vi "ni_move.vi"(6 "Axis enable":bool[](array[boolean])=[TRUE, TRUE, TRUE, TRUE], 8 "error in":errorcluster, 9 "Axis positions":dbl[](array[numeric])=[0.0, 0.0, 0.0, 0.0], 10 "Absolute":bool=TRUE) -> (0 "error out":errorcluster)   [LabVIEW 2011]
uses:
  <vilib>/Motion/FlexMotion/CustomControls/CustomControls.llb/AxisOrVectorSpaceControl To Control.flx
  <vilib>/Motion/FlexMotion/CustomControls/CustomControls.llb/AxisOrVectorSpace To Configure.flx
  <vilib>/Motion/FlexMotion/FunctionsVIs/StartStopMotion.llb/Start Motion (8 axes).flx
  <vilib>/Motion/FlexMotion/FunctionsVIs/Trajectory.llb/Wait for Move Complete (8 axes).flx
panel:
  in  "Timeout":u32=60000
  # "The purposes of axis enable is to allow a subset of axes to be driven in absolute position mode without changing (or knowing) the positions of the other axes.   Being disabled just means that we don't want to move that axis, not that we want it powered down."
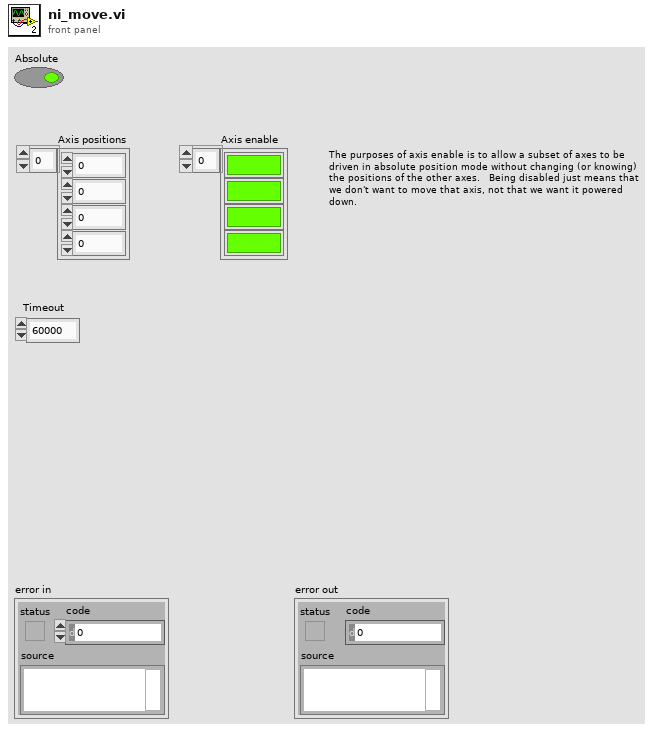
[diagram p1: front panel]
types:
  T1 = typedef "Board Id" = u8
  T2 = enum16{"Absolute Position", "Relative Position", "Velocity", "Relative to Cap Pos", "Modulus Position", "Absolute Contouring", "Relative Contouring"}
  T3 = typedef "AxisOrVectorSpaceControl To Control.flx" = u16
  T4 = typedef "AxisOrVectorSpace To Configure.flx" = u16
  T5 = typedef "Resource Out (Enum).flx" = u16
  T6 = typedef "Bd Id Out" = u8
  T7 = cluster{"Axis enable[0]":bool, "Axis enable[1]":bool, "Axis enable[2]":bool, "Axis enable[3]":bool, "Axis enable[4]":bool, "Axis enable[5]":bool, "Axis enable[6]":bool, "Axis enable[7]":bool}
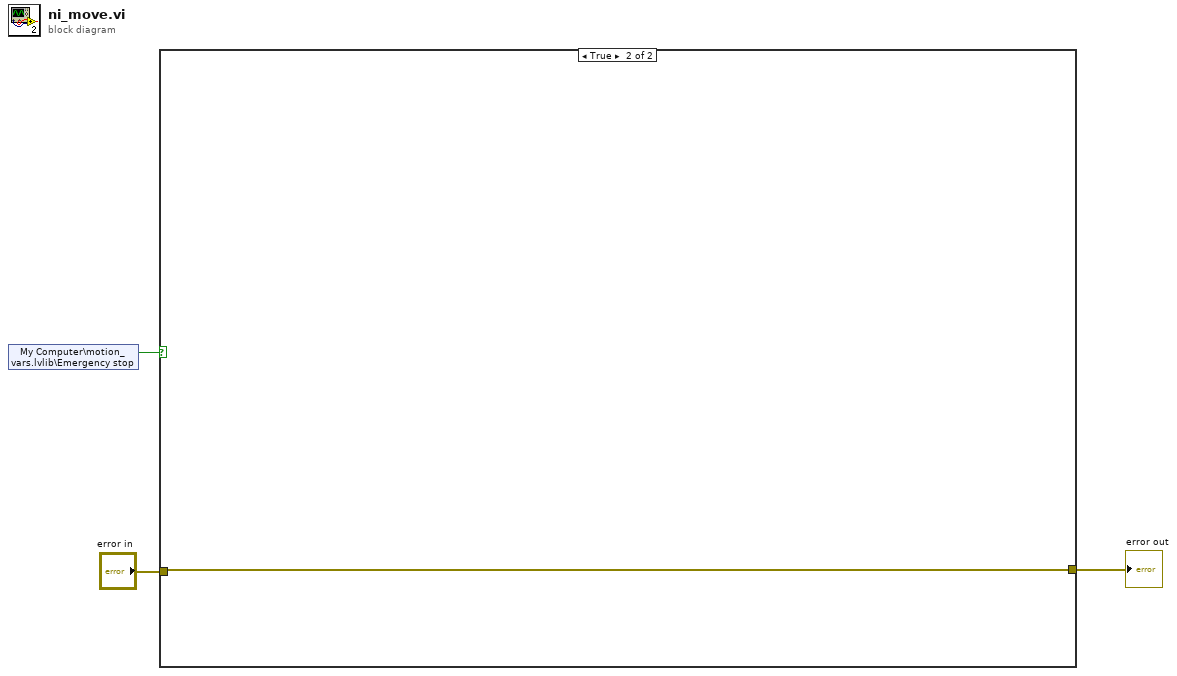
[diagram p0: block diagram]
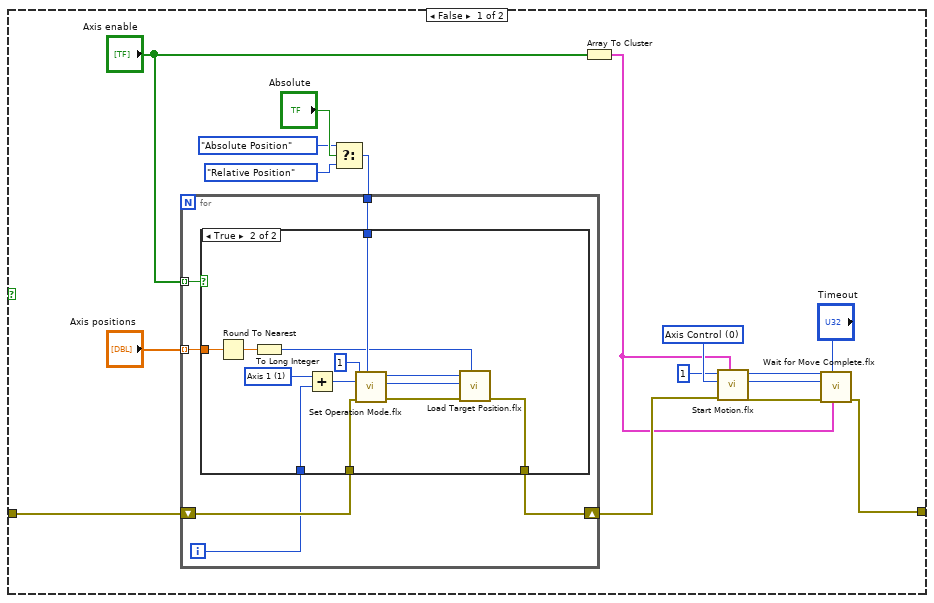
[diagram p2: hidden frame]
diagram:
  n1 = shared-variable "My Computer\\motion_vars.lvlib\\Emergency stop"() -> (w1:bool)  [unwired: 1 in, 1 out]
  n2 = case shown="True" w1 {
    tunnel: "error in" -> [w18 w40]
    tunnel: [w7 w40] -> w2
    frame False {
      w11 = T3 0 items=["Axis Control"=0, "Axis 1"=1, "Axis 2"=2, "Axis 3"=3, "Axis 4"=4, "Axis 5"=5, "Axis 6"=6, "Axis 7"=7, "Axis 8"=8, "Vector Space Control"=16, "Vector Space 1"=17, "Vector Space 2"=18, "Vector Space 3"=19, "Vector Space 4"=20] ("Axis or Vector Space")
      n3 = Select(t=T2."Absolute Position" ("Position Mode (Absolute)"), s="Absolute", f=T2."Relative Position" ("Position Mode (Absolute)")) -> (s? t:f=w15:T2)
      n4 = for {
        tunnel: "Axis enable" -> [w23] mode=indexing
        tunnel: "Axis positions" -> [w22] mode=indexing
        shift-right: [w21] -> w12
        shift-left: w18 -> [w25]
        tunnel: w15 -> [w24]
        i -> [w20]
        n5 = case shown="True" w23 {
          tunnel: w25 -> [w26 w37]
          tunnel: w20 -> [_ w36]
          tunnel: w24 -> [_ w35]
          tunnel: w22 -> [_ w31]
          tunnel: [w26 w28] -> w21
          frame False {
          }
          frame True {
            w39 = T4 1 items=["Axis 1"=1, "Axis 2"=2, "Axis 3"=3, "Axis 4"=4, "Axis 5"=5, "Axis 6"=6, "Axis 7"=7, "Axis 8"=8, "Vector Space 1"=17, "Vector Space 2"=18, "Vector Space 3"=19, "Vector Space 4"=20] ("Axis or Vector Space")
            n6 = Round To Nearest(number=w31) -> (nearest integer value=w30:dbl)
            n7 = To Long Integer(number=w30) -> (32bit integer=w29:i32)
            n8 = Add(x=w39, y=w36) -> (x+y=w38:i32)
            n9 = call <vilib>:"Set Operation Mode.flx"("Position Mode (Absolute)"=w35, "error in (no error)"=w37, "Axis or Vector Space"=w38, "Board ID"=T1 1) -> ("error out"=w32:errorcluster, "Resource Output"=w33:T5, "Bd ID Out"=w34:T6)  [unwired: 2 in]
            n10 = call <vilib>:"Load Target Position.flx"("Target Position (0)"=w29, "error in (no error)"=w32, "Axis"=w33, "Board ID"=w34) -> ("error out"=w28:errorcluster)  [unwired: 3 in, 2 out]
          }
        }
      }
      n11 = Array To Cluster(array="Axis enable") -> (cluster=w10:T7)
      n12 = call-poly <vilib>:"Start Motion.flx"("Axis/VS Map (Disabled)"=w10, "error in (no error)"=w12, "Axis or Vector Space"=w11, "Board ID"=T1 1) -> ("error out"=w8:errorcluster, "Resource Output"=w9:T5, "Bd ID Out"=w5:T6)  [unwired: 2 in]
      n13 = call-poly <vilib>:"Wait for Move Complete.flx"("Axis/VS Map (Disabled)"=w10, "Timeout (10000 ms)"="Timeout", "error in (no error)"=w8, "Axis or Vector Space"=w9, "Board ID"=w5) -> ("error out"=w7:errorcluster)  [unwired: 3 in, 3 out]
    }
    frame True {
    }
  }
  "error out" <- w2
